vi "GDSProject_GetProjects.vi"(1 "GetProjectRefByName":string, 5 "error in (no error)":errorcluster, 7 "OpenProjectRef(True)":bool=TRUE) -> (15 "Projects":string[](array[string]), 16 "Project Refnum":refnum<vi>, 19 "error out":errorcluster)   [LabVIEW 2016]
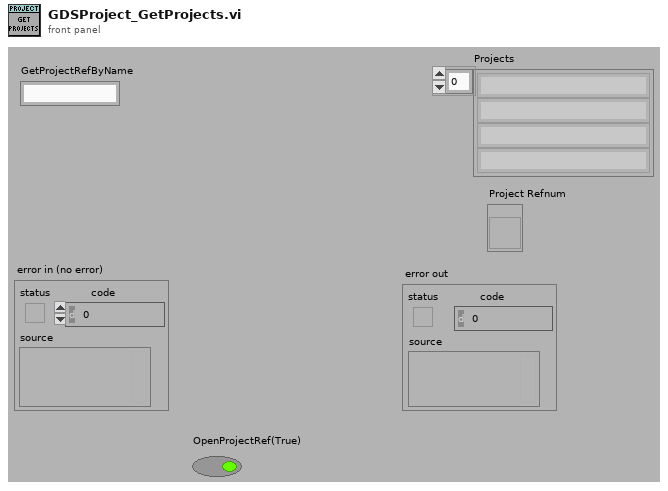
[diagram p1: front panel]
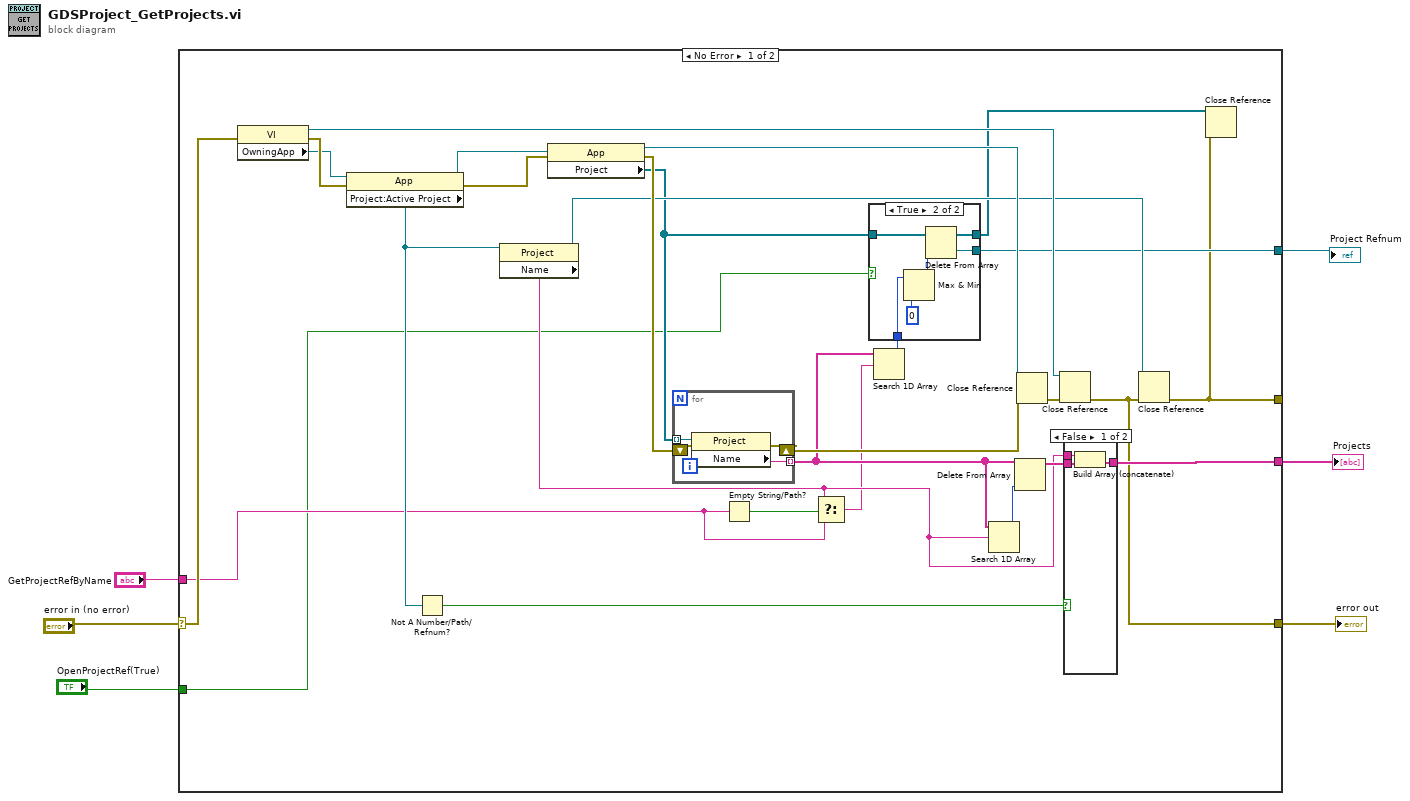
[diagram p0: block diagram]
diagram:
  n1 = case shown="No Error" "error in (no error)" {
    selector: "error in (no error)" -> [w34 w50]
    tunnel: [w18 w50] -> w5
    tunnel: [w24 _] -> w4
    tunnel: "GetProjectRefByName" -> [w11 _]
    tunnel: [w19 _] -> w2
    tunnel: [w8 _] -> _
    tunnel: "OpenProjectRef(True)" -> [w7 _]
    frame No Error {
      n2 = property class="VI"(error in=w34) -> (reference out=w31:refnum<vi>, error out=w30:errorcluster, "OwningApp"=w29:refnum<vi>)  [unwired: 1 in]
      n3 = property class="App"(reference=w29, error in=w30) -> (reference out=w28:refnum<vi>, error out=w27:errorcluster, "Project:Active Project"=w17:refnum<vi>)
      n4 = Not A Number/Path/Refnum?(number/path/refnum=w17) -> (NaN/Path/Refnum?=w16:bool)
      n5 = property class="Project"(reference=w17) -> (reference out=w21:refnum<vi>, "Name"=w12:string)  [unwired: 1 in, 1 out]
      n6 = property class="App"(reference=w28, error in=w27) -> (reference out=w33:refnum<vi>, error out=w23:errorcluster, "Project"=w20:refnum<vi>[])
      n7 = for {
        tunnel: w20 -> [w45] mode=indexing
        tunnel: [w43] -> w14 mode=indexing
        shift-right: [w42] -> w22
        shift-left: w23 -> [w44]
        n8 = property class="Project"(reference=w45, error in=w44) -> (error out=w42:errorcluster, "Name"=w43:string)  [unwired: 1 out]
      }
      n9 = Empty String/Path?(string/path=w11) -> (empty?=w13:bool)
      n10 = Select(t=w12, s=w13, f=w11) -> (s? t:f=w10:string)
      n11 = Search 1D Array(1D array=w14, element=w10) -> (index of element=w9:i32)  [unwired: 1 in]
      n12 = case shown="True" w7 {
        tunnel: w20 -> [w35 w41]
        tunnel: [_ w40] -> w19
        tunnel: [w35 w39] -> w15
        tunnel: w9 -> [_ w37]
        frame False {
        }
        frame True {
          n13 = Max & Min(x=w37, y=0) -> (max(x,y)=w36:i32)  [unwired: 1 out]
          n14 = Delete From Array(array=w41, index=w36) -> (deleted portion=w40:refnum<vi>, array with subset deleted=w39:refnum<vi>[])  [unwired: 1 in]
        }
      }
      n15 = Search 1D Array(1D array=w14, element=w12) -> (index of element=w26:i32)  [unwired: 1 in]
      n16 = Delete From Array(array=w14, index=w26) -> (array with subset deleted=w25:string[])  [unwired: 1 in, 1 out]
      n17 = Close Reference(reference=w33, error in (no error)=w22) -> (error out=w32:errorcluster)
      n18 = Close Reference(reference=w31, error in (no error)=w32) -> (error out=w18:errorcluster)
      n19 = case shown="False" w16 {
        tunnel: w25 -> [w48 w49]
        tunnel: w12 -> [w47 _]
        tunnel: [w46 w49] -> w24
        frame False {
          n20 = Build Array (concatenate)(w47, w48) -> (w46:string[])
        }
        frame True {
        }
      }
      n21 = Close Reference(reference=w21, error in (no error)=w18) -> (error out=w8:errorcluster)
      n22 = Close Reference(reference=w15, error in (no error)=w8) -> ()  [unwired: 1 out]
    }
    frame Error {
    }
  }
  "error out" <- w5
  "Projects" <- w4
  "Project Refnum" <- w2
